vi "Adjust Slit (1).vi"(8 "error in (no error)":errorcluster, 10 "SLIT WIDTH":dbl[unit]=5.0000000000000016e-05 min=0.0 max=0.005000000000000002 step=1.0000000000000004e-06, 11 "VISA resource name":refnum<visa-resource-name>) -> (0 "error out":errorcluster, 3 "VISA resource name out":refnum<visa-resource-name>)   [LabVIEW 2017, in "Digikrom DK24x.lvlib"]
doc: "Adjusts entrance slit to a given width."
uses:
  Digikrom DK24x.lvlib
  Private/Command.ctl
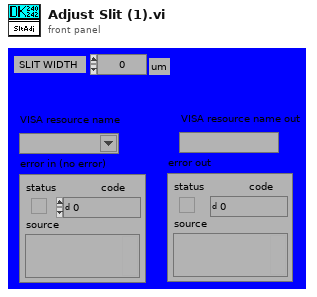
[diagram p1: front panel]
types:
  T1 = typedef "Digikrom DK24x.lvlib/Command.ctl" = u8
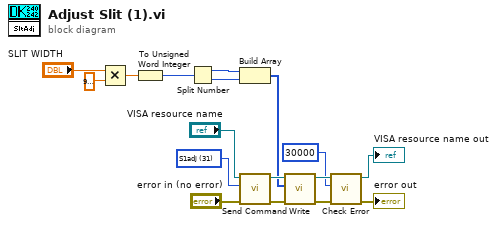
[diagram p0: block diagram]
diagram:
  w1 = T1 31 items=["Cancel"=24, "Clear"=25, "CSR"=28, "Echo"=27, "Filter"=15, "Gcal"=18, "Goto"=16, "Grtid?"=19, "Grtsel"=26, "NOVRAM Read"=56, "NOVRAM Write"=59, "Reset"=255, "Scan"=12, "Scan Up"=9, "Scan Down"=3, "Serial?"=33, "Slew Up"=8, "Slew Down"=2, "Slit Reset"=43, "Slit?"=30, "Sltadj"=14, "Speed"=13, "Sspeed?"=21, "Step Down"=1, "Step Up"=7, "S1adj"=31, "S2adj"=32, "S3adj"=34, "S1cal"=22, "S2cal"=23, "S3cal"=35, "Test"=17, "Type"=57, "Wave?"=29, "Zero"=52] ("Command")
  n1 = Multiply(x="SLIT WIDTH", y=dbl[unit] 999999.9999999995 ("/um")) -> (x*y=w16:dbl)
  n2 = To Unsigned Word Integer(number=w16) -> (unsigned 16bit integer=w17:u16)
  n3 = Split Number(x=w17) -> (hi(x)=w13:u8, lo(x)=w14:u8)
  n4 = Build Array(w13, w14) -> (w2:u8[])
  n5 = call "Send Command.vi"("error in (no error)"="error in (no error)", "Command"=w1, "VISA resource name"="VISA resource name") -> ("error out"=w11:errorcluster, "VISA resource name out"=w12:refnum<visa-resource-name>)  [unwired: 7 out]
  n6 = call "Write.vi"("error in (no error)"=w11, "Byte Array"=w2, "VISA resource name"=w12) -> ("error out"=w9:errorcluster, "VISA resource name out"=w10:refnum<visa-resource-name>)  [unwired: 7 out]
  n7 = call "Check Error.vi"("error in"=w9, "timeout"=u32 30000, "VISA resource name in"=w10) -> ("error out"=→"error out":errorcluster, "VISA resource name out"=→"VISA resource name out":refnum<visa-resource-name>)  [unwired: 7 out]
